vi "Radau5_Matrix JM.vi"(9 "Step size":dbl, 10 "Matrix M":T2, 11 "Matrix J":T2) -> (2 "Inverse of Matrix JM_2":T1, 3 "Inverse of Matrix JM_1":T2)   [LabVIEW 2017, in "NI_DAE.lvlib"]
uses:
  <vilib>/gmath/NI_DAE.lvlib
  <vilib>/Analysis/Matrix/Datatypes/RealMatrix.ctl
  <vilib>/Analysis/Matrix/Datatypes/ComplexMatrix.ctl
  <vilib>/Analysis/Matrix/Numeric/Complex/Cartesian To Complex - RM,R.vi
  <vilib>/Analysis/Matrix/Numeric/Multiply/Multiply - RM,R.vi
  <vilib>/Analysis/Matrix/Numeric/Add/Add - RM,RM.vi
  <vilib>/Analysis/baseanly.llb/Real Inverse Matrix.vi
  <vilib>/Analysis/Matrix/Numeric/Multiply/Multiply - CM,C.vi
  <vilib>/Analysis/Matrix/Numeric/Add/Add - CM,CM.vi
  <vilib>/Analysis/baseanly.llb/Complex Inverse Matrix.vi
  <vilib>/Analysis/Matrix/NI_Matrix.lvlib
  <vilib>/Analysis/NI_AALBase.lvlib
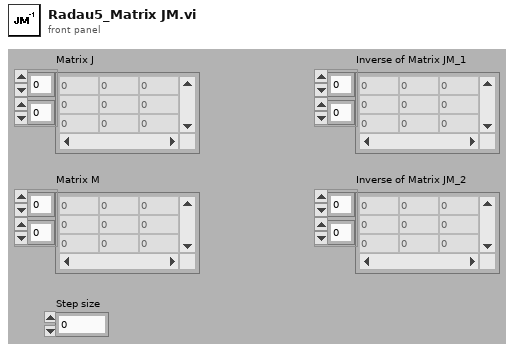
[diagram p1: front panel]
types:
  T1 = typedef "NI_Matrix.lvlib/ComplexMatrix.ctl" = cdb[][]
  T2 = typedef "NI_Matrix.lvlib/RealMatrix.ctl" = dbl[][]
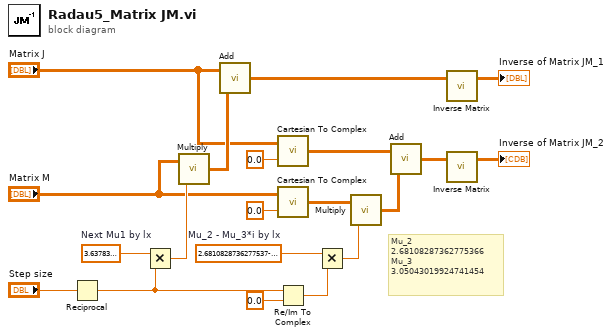
[diagram p0: block diagram]
diagram:
  w1 = cdb 2.6810828736277537-3.0504301992474145i  # Mu_2 - Mu_3*i by lx
  w5 = 3.637834252744496  # Next Mu1 by lx
  # "Mu_2\n2.68108287362775366\nMu_3\n3.05043019924741454"
  n1 = Reciprocal(x="Step size") -> (1/x=w14:dbl)
  n2 = Multiply(x=w5, y=w14) -> (x*y=w20:dbl)
  n3 = call-poly <vilib>:"Multiply.vi"("Real Scalar c"=w20, "Real Matrix A"="Matrix M") -> ("A * c"=w19:T2)
  n4 = call-poly <vilib>:"Add.vi"("Real Matrix B"=w19, "Real Matrix A"="Matrix J") -> ("A + B"=w18:T2)
  n5 = call-poly <vilib>:"Cartesian To Complex.vi"("Real Scalar k"=0.0, "Real Matrix R"="Matrix J") -> ("R + ki"=w8:T1)
  n6 = call-poly <vilib>:"Cartesian To Complex.vi"("Real Scalar k"=0.0, "Real Matrix R"="Matrix M") -> ("R + ki"=w11:T1)
  n7 = Re/Im To Complex(1:0.0 ("y"), 2:w14) -> (0:w13:cdb)
  n8 = Multiply(x=w1, y=w13) -> (x*y=w16:cdb)
  n9 = call-poly <vilib>:"Multiply.vi"("Complex Scalar c"=w16, "Complex Matrix A"=w11) -> ("A * c"=w10:T1)
  n10 = call-poly <vilib>:"Add.vi"("Complex Matrix B"=w10, "Complex Matrix A"=w8) -> ("A + B"=w7:T1)
  n11 = call-poly <vilib>:"Inverse Matrix.vi"("Input Matrix"=w18) -> ("Inverse Matrix"=→"Inverse of Matrix JM_1":T2)  [unwired: 1 in, 1 out]
  n12 = call-poly <vilib>:"Inverse Matrix.vi"("Input Matrix"=w7) -> ("Inverse Matrix"=→"Inverse of Matrix JM_2":T1)  [unwired: 1 in, 1 out]
